vi "Disconnect.vi"(8 "error in (no error)":errorcluster, 10 "Disconnection list in":string, 11 "NI-SWITCH Consumer in":refnum<class "NI-SWITCH Consumer.lvclass">) -> (0 "error out":errorcluster, 3 "NI-SWITCH Consumer out":refnum<class "NI-SWITCH Consumer.lvclass">)   [LabVIEW 2020, in "NI-SWITCH Messaging.lvlib" / "NI-SWITCH Consumer.lvclass"]
uses:
  NI-SWITCH Consumer.lvclass
  NI-SWITCH Consumer.lvclass/NI-SWITCH Consumer.ctl
  <instrlib>/niSwitch/niSwitch.llb/niSwitch Disconnect Channels (Multiple).vi
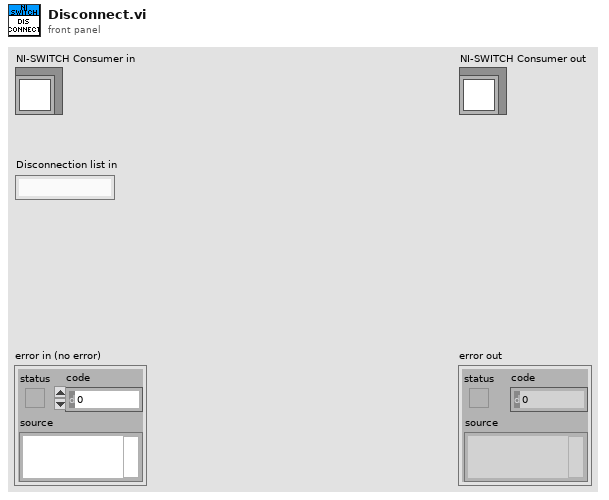
[diagram p1: front panel]
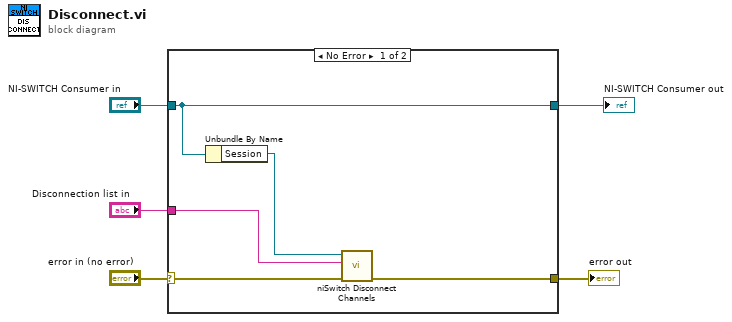
[diagram p0: block diagram]
diagram:
  n1 = case shown="No Error" "error in (no error)" {
    selector: "error in (no error)" -> [w7 w12]
    tunnel: [w6 w12] -> w3
    tunnel: [w10 w11] -> w2
    tunnel: "NI-SWITCH Consumer in" -> [w10 w11]
    tunnel: "Disconnection list in" -> [w9 _]
    frame No Error {
      n2 = Unbundle By Name(w10) -> ("Session"=w8:refnum<k15>)
      n3 = call-poly <instrlib>:"niSwitch Disconnect Channels.vi"("error in (no error)"=w7, "disconnection list"=w9, "instrument handle"=w8) -> ("error out"=w6:errorcluster)  [unwired: 7 in, 1 out]
    }
    frame Error {
    }
  }
  "error out" <- w3
  "NI-SWITCH Consumer out" <- w2
